vi "LabVIEW+Suite Demo Station.vi"() -> ()   [LabVIEW 2020]
doc: "This template is for the Queued Message Handler design pattern.\n\nThe Event Handling Loop generates messages based on user interface actions.\n\nThe Message Handling Loop processes messages generated by the Event Handling Loop, or by other messages. The messages are string values, so new messages can be added easily to the Message Cases case structure in the Message Handling Loop. Each message cluster can also provide an optional value for Message Data, which is a variant that can be converted to whatever message-specific data is required."
uses:
  support/Demo_class/Demo.lvclass
  support/Demo_class/Demo.lvclass/Demo.ctl
  support/UI Data--cluster.ctl
  support/Message Queue/lvdemo_Message Queue.lvlib
  support/Message Queue/Enqueue Message (Single).vi
  support/Configuration--cluster.ctl
  support/Tree Tag to Demo--map.ctl
panel:
  out "Title Text":string
  in  "Favorites Ring":u16(ring) items=["All Features"]
  in  "Tree":string(tree)
  in  "Slideshow":bool
  in  "Back":bool
  in  "Try It":bool
  in  "Credits":string="The code for this demo station is available at bit.ly/labviewdemostation"
  in  "Forward":bool
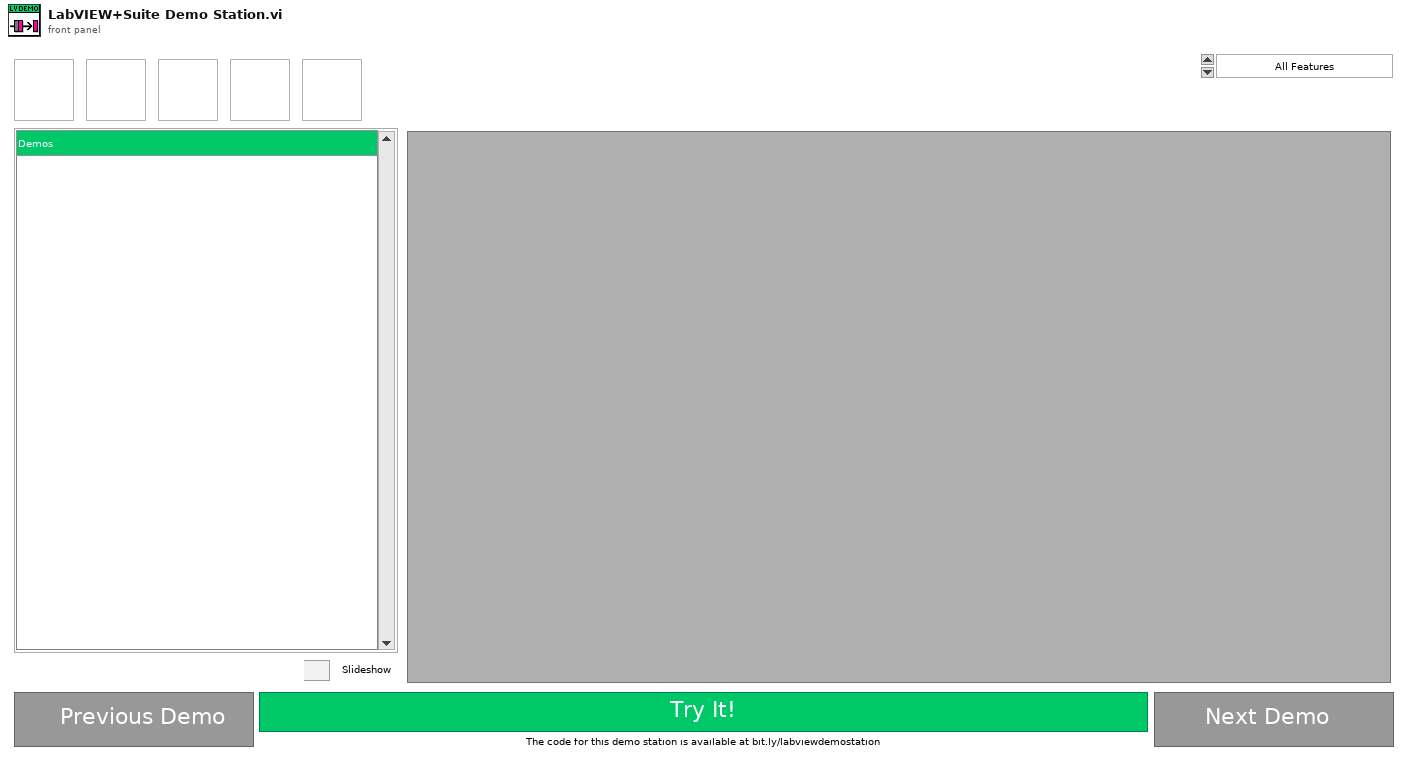
[diagram p1: front panel]
types:
  T1 = typedef "UI Data--cluster.ctl" = cluster{"Configuration":T2, "Start Timestamp":dbl, "Active Demos":T3, "Available Demos":T3}
  T2 = typedef "Configuration--cluster.ctl" = cluster{"Window Title":string, "Start Maximized":bool, "Slide Duration":i32, "Ignored Demos":string[], "Top Level Folder Order":string[], "Favorites":map{string, string[]}}
  T3 = typedef "Tree Tag to Demo--map.ctl" = map{string, refnum<class "Demo.lvclass">}
  T4 = typedef "lvdemo_Message Queue.lvlib/All Message Queues.ctl" = cluster{"UI":refnum<queue>}
  T5 = typedef "eventvkey.ctl" = enum16{"ASCII", "Enter", "Return", "Shift", "Ctrl", "Alt", "Cmd", "Opt", "Caps", "NumLock", "Clear", "Break", "Up", "Down", "Left", "Right", "Insert", "Delete", "Home", "End", "PageUp", "PageDown", "Escape", "Help", "Pause", "ScrollLock", "F1", "F2", "F3", "F4", "F5", "F6", "F7", "F8", "F9", "F10", "F11", "F12", "F13", "F14", "F15", "F16", "F17", "F18", "F19", "F20", "F21", "F22", "F23", "F24", "Play", "VolumeUp", "VolumeDown", "Mute", "Two Byte Char"}
  T6 = enum32{"Invalid", "Standard", "Closed", "Hidden", "Minimized", "Maximized"}
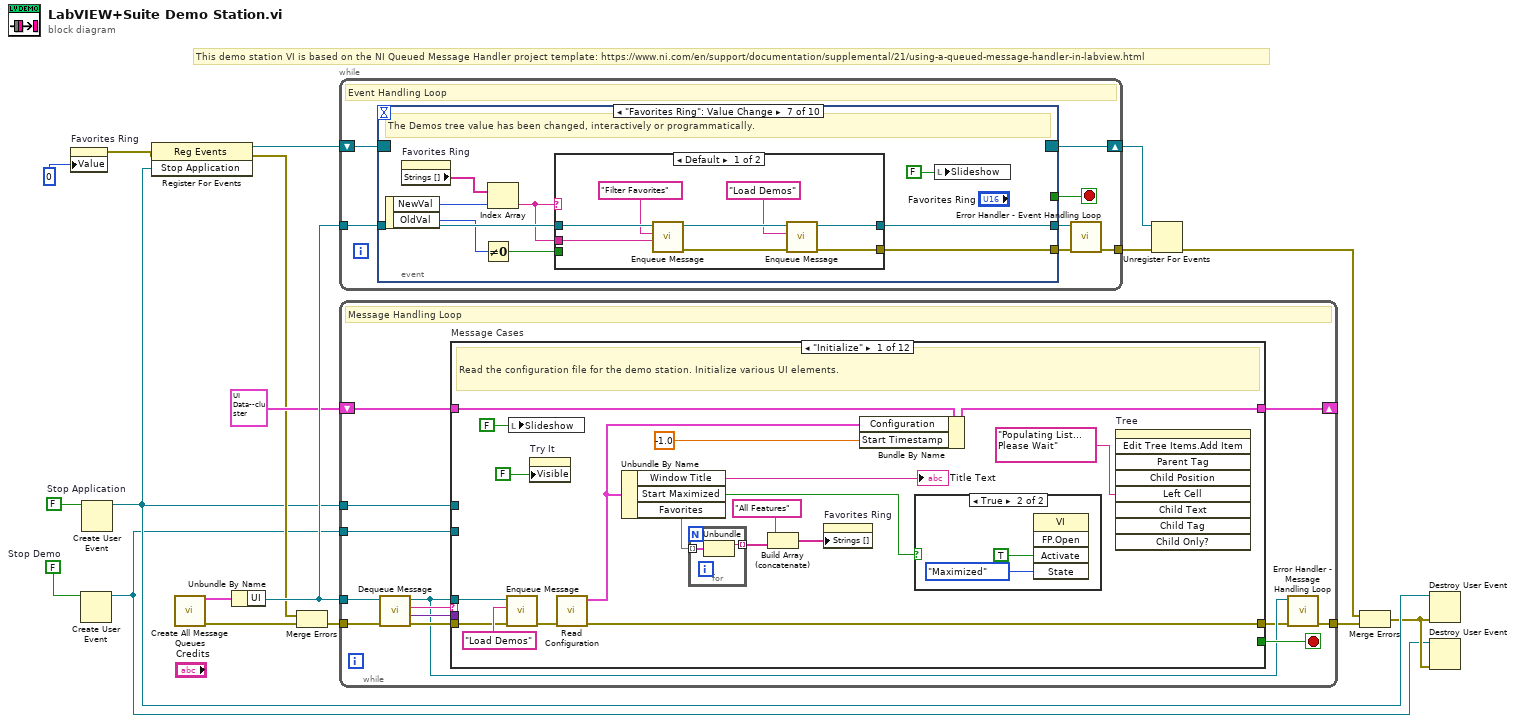
[diagram p0: block diagram]
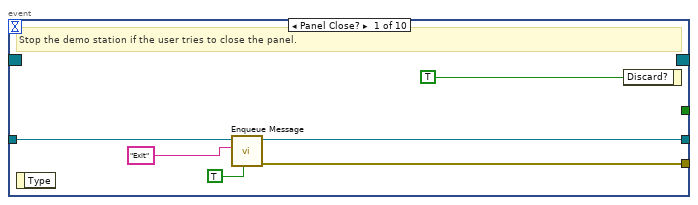
[diagram p2: hidden frame]
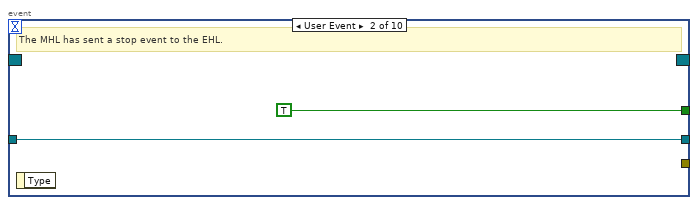
[diagram p3: hidden frame]
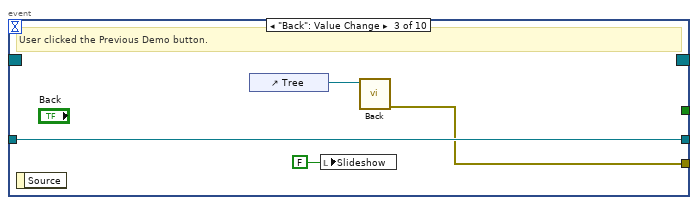
[diagram p4: hidden frame]
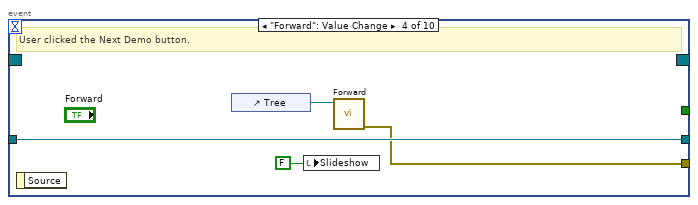
[diagram p5: hidden frame]
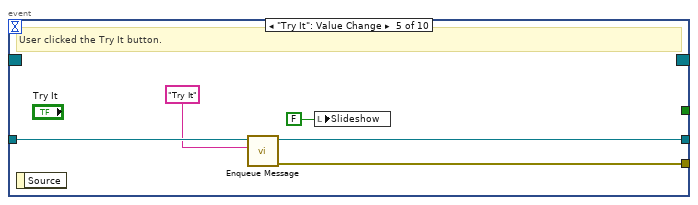
[diagram p6: hidden frame]
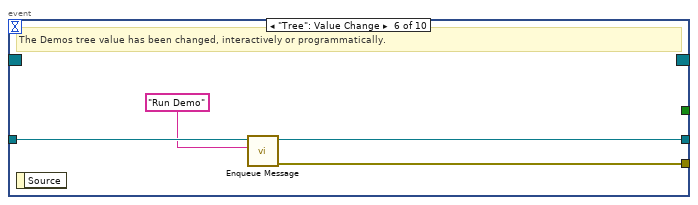
[diagram p7: hidden frame]
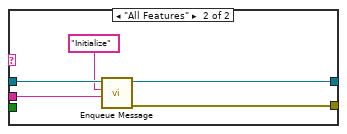
[diagram p8: hidden frame]
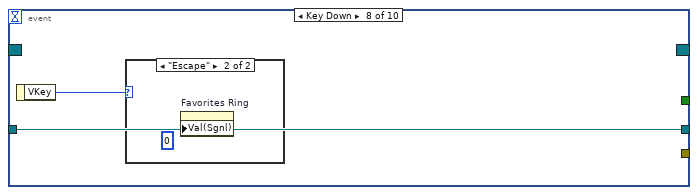
[diagram p9: hidden frame]
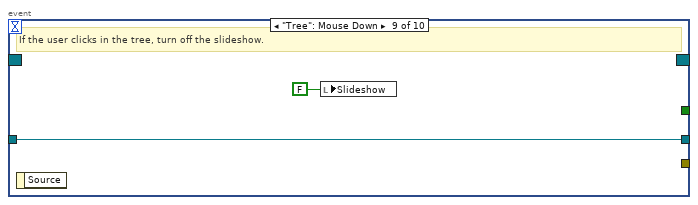
[diagram p11: hidden frame]
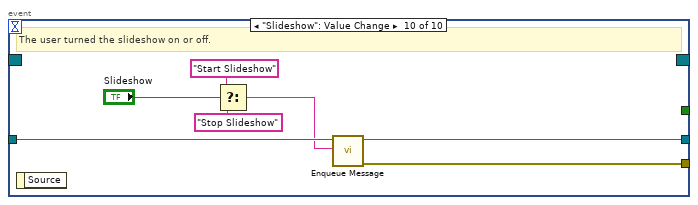
[diagram p12: hidden frame]
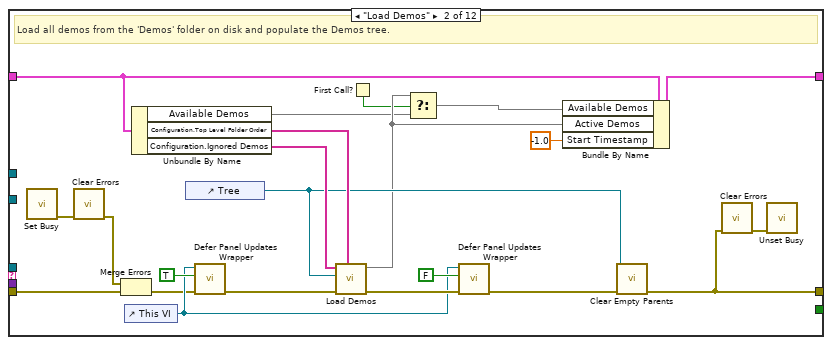
[diagram p14: hidden frame]
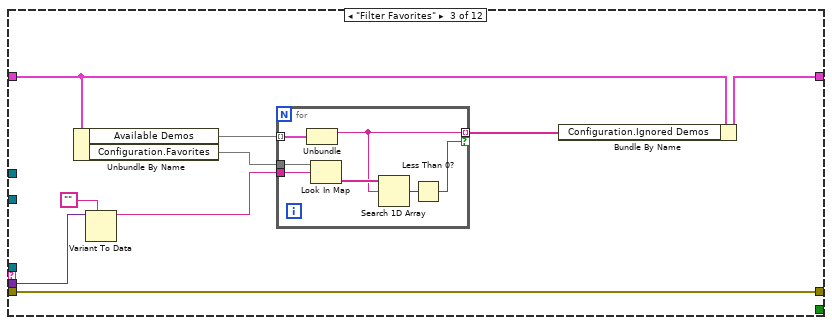
[diagram p15: hidden frame]
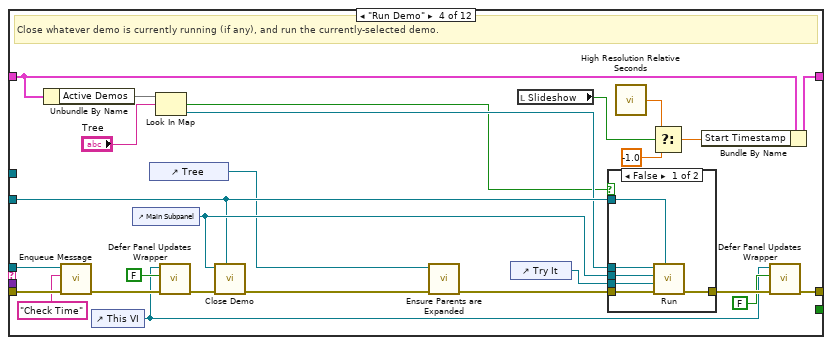
[diagram p16: hidden frame]
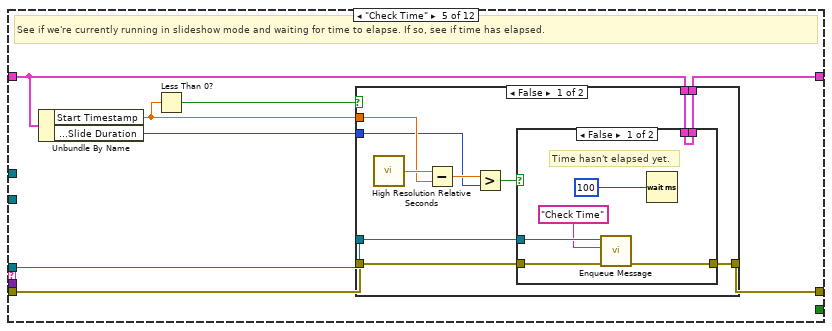
[diagram p18: hidden frame]
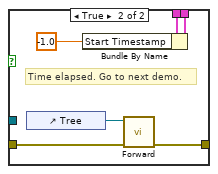
[diagram p19: hidden frame]
diagram:
  w5 = FALSE  # Stop Demo
  w7 = FALSE  # Stop Application
  # "This demo station VI is based on the NI Queued Message Handler project template: https://www.ni.com/en/support/documentation/supplemental/21/using-a-queued-message-handler-in-labview.html"
  n1 = property on="Favorites Ring" class="Ring (strict)"("Value"=u16 0 ("Value (Signaling)")) -> (error out=w1:errorcluster)  [unwired: 2 in, 1 out]
  n2 = Create User Event(user event datatype=w5) -> (user event=w3:refnum<user-event>)  [unwired: 1 in, 1 out]
  n3 = Create User Event(user event datatype=w7) -> (user event=w6:refnum<user-event>)  [unwired: 1 in, 1 out]
  n4 = register-events(error in=w1, w6) -> (reference out=w10:refnum<event-registration>, error out=w8:errorcluster)  [unwired: 1 in]
  n5 = call "Create All Message Queues.vi"() -> ("error out"=w18:errorcluster, "Message Queues out"=w17:T4)  [unwired: 10 in]
  n6 = Unbundle By Name(w17) -> ("UI"=w15:refnum<queue>)
  n7 = Merge Errors(w8, w18) -> (w9:errorcluster)
  n8 = while {
    tunnel: w15 -> [w25]
    shift-right: [w23] -> w13
    shift-left: w10 -> [w24]
    tunnel: [w19] -> w11
    stop <- w21 stop-if-true
    # "Event Handling Loop"
    n9 = event shown="[6] \"Favorites Ring\": Value Change" {
      selector: w24 -> [_ _ _ _ _ _ _ _ _ _]
      dyn-events: [_ _ _ _ _ _ _ _ _ _] -> w23
      timeout: _ -> [_ _ _ _ _ _ _ _ _ _]
      tunnel: [_ TRUE ("Discard?") _ _ _ _ _ _ _ _] -> w21
      tunnel: w25 -> [w30 w33 w37 w41 w46 w50 w59 w74 w77 w84]
      tunnel: [w29 _ w35 w39 w44 w48 w58 _ _ w80] -> w22
      tunnel: [w28 w33 w37 w41 w45 w49 w57 w74 w77 w81] -> w20
      event Panel Close? {
        # "Stop the demo station if the user tries to close the panel."
        n10 = event-data() -> ()  [unwired: 1 in, 1 out]
        n11 = call-poly "Enqueue Message.vi"("Priority Message? (F)"=TRUE, "Message"="Exit", "Message Queue"=w30) -> ("error out"=w29:errorcluster, "dup Message Queue"=w28:refnum<queue>)  [unwired: 7 in]
        n12 = event-data("Discard?"=TRUE) -> ()  [unwired: 1 in, 1 out]
      }
      event User Event {
        # "The MHL has sent a stop event to the EHL."
        n13 = event-data() -> ()  [unwired: 1 in, 1 out]
      }
      event "Back": Value Change {
        # "User clicked the Previous Demo button."
        n14 = event-data() -> ()  [unwired: 1 in, 1 out]
        n15 = control-ref of="Tree"() -> (w36:refnum<vi>)
        n16 = local write "Slideshow"(FALSE ("Slideshow")) -> ()
        n17 = call "Back.vi"("Tree"=w36) -> ("error out"=w35:errorcluster)  [unwired: 10 in]
      }
      event "Forward": Value Change {
        # "User clicked the Next Demo button."
        n18 = event-data() -> ()  [unwired: 1 in, 1 out]
        n19 = control-ref of="Tree"() -> (w40:refnum<vi>)
        n20 = local write "Slideshow"(FALSE ("Slideshow")) -> ()
        n21 = call "Forward.vi"("Tree"=w40) -> ("error out"=w39:errorcluster)  [unwired: 10 in]
      }
      event "Try It": Value Change {
        # "User clicked the Try It button."
        n22 = event-data() -> ()  [unwired: 1 in, 1 out]
        n23 = call-poly "Enqueue Message.vi"("Message"="Try It", "Message Queue"=w46) -> ("error out"=w44:errorcluster, "dup Message Queue"=w45:refnum<queue>)  [unwired: 8 in]
        n24 = local write "Slideshow"(FALSE ("Slideshow")) -> ()
      }
      event "Tree": Value Change {
        # "The Demos tree value has been changed, interactively or programmatically."
        n25 = event-data() -> ()  [unwired: 1 in, 1 out]
        n26 = call-poly "Enqueue Message.vi"("Message"="Run Demo", "Message Queue"=w50) -> ("error out"=w48:errorcluster, "dup Message Queue"=w49:refnum<queue>)  [unwired: 8 in]
      }
      event "Favorites Ring": Value Change {
        # "The Demos tree value has been changed, interactively or programmatically."
        n27 = event-data() -> ("NewVal"=w54:u16, "OldVal"=w52:u16)  [unwired: 1 in]
        n28 = property on="Favorites Ring" class="Ring (strict)"() -> ("Strings []"=w55:string[])  [unwired: 2 in, 2 out]
        n29 = Not Equal To 0?(x=w52) -> (x != 0?=w51:bool)
        n30 = Index Array(array=w55, index=w54) -> (element=w53:string)
        n31 = case shown="Default" w53 {
          tunnel: w59 -> [w61 w72]
          tunnel: [w65 w69] -> w58
          tunnel: [w64 w70] -> w57
          tunnel: w53 -> [w62 w68]
          tunnel: w51 -> [_ _]
          frame Default {
            n32 = call-poly "Enqueue Message.vi"("Message Data"=w62, "Message"="Filter Favorites", "Message Queue"=w61) -> ("error out"=w66:errorcluster, "dup Message Queue"=w67:refnum<queue>)  [unwired: 7 in]
            n33 = call-poly "Enqueue Message.vi"("error in (no error)"=w66, "Message"="Load Demos", "Message Queue"=w67) -> ("error out"=w65:errorcluster, "dup Message Queue"=w64:refnum<queue>)  [unwired: 7 in]
          }
          frame "All Features" {
            n34 = call-poly "Enqueue Message.vi"("Message Data"=w68, "Message"="Initialize", "Message Queue"=w72) -> ("error out"=w69:errorcluster, "dup Message Queue"=w70:refnum<queue>)  [unwired: 7 in]
          }
        }
        n35 = local write "Slideshow"(FALSE ("Slideshow")) -> ()
      }
      event Key Down {
        n36 = event-data() -> ("VKey"=w73:T5)  [unwired: 1 in]
        n37 = case shown="\"Escape\"" w73 {
          frame "ASCII", Default {
          }
          frame "Escape" {
            n38 = property on="Favorites Ring" class="Ring (strict)"("Val(Sgnl)"=u16 0 ("Value (Signaling)")) -> ()  [unwired: 2 in, 2 out]
          }
        }
      }
      event "Tree": Mouse Down {
        # "If the user clicks in the tree, turn off the slideshow."
        n39 = event-data() -> ()  [unwired: 1 in, 1 out]
        n40 = local write "Slideshow"(FALSE ("Slideshow")) -> ()
      }
      event "Slideshow": Value Change {
        # "The user turned the slideshow on or off."
        n41 = event-data() -> ()  [unwired: 1 in, 1 out]
        n42 = Select(t="Start Slideshow", s="Slideshow", f="Stop Slideshow") -> (s? t:f=w78:string)
        n43 = call-poly "Enqueue Message.vi"("Message"=w78, "Message Queue"=w84) -> ("error out"=w80:errorcluster, "dup Message Queue"=w81:refnum<queue>)  [unwired: 8 in]
      }
    }
    n44 = call "Error Handler - Event Handling Loop.vi"("error in (no error)"=w22, "Message Queue"=w20) -> ("dup error in"=w19:errorcluster)  [unwired: 8 in, 1 out]
  }
  n45 = while {
    tunnel: w15 -> [w89]
    shift-right: [w96] -> _
    shift-left: T1 {"Configuration"={"Window Title"="", "Start Maximized"=FALSE, "Slide Duration"=0, "Ignored Demos"=[], "Top Level Folder Order"=[], "Favorites"={}}, "Start Timestamp"=0.0, "Active Demos"={}, "Available Demos"={}} ("Data Cluster") -> [w97]
    tunnel: w6 -> [w94]
    tunnel: w9 -> [w93]
    tunnel: [w87] -> w16
    tunnel: w3 -> [w85]
    stop <- w95 stop-if-true
    # "Message Handling Loop"
    n46 = call "Dequeue Message.vi"("error in (no error)"=w93, "Message Queue"=w89) -> ("error out"=w92:errorcluster, "Message Data"=w90:variant, "Message"=w91:string, "dup Message Queue"=w88:refnum<queue>)  [unwired: 6 in]
    n47 = case "Message Cases" shown="\"Initialize\"" w91 {
      selector: w91 -> [_ _ _ _ _ _ _ _ _ _ _ w277]
      tunnel: w88 -> [w110 _ _ w182 w195 _ _ _ _ _ w270 _]
      tunnel: w92 -> [w108 w138 w150 w183 w194 w226 w235 w241 w248 w251 w266 _]
      tunnel: [w106 w125 w150 w169 w193 w227 w234 w241 w242 w249 w267 w274] -> w86
      tunnel: w97 -> [w115 w127 w149 w178 w191 w230 w236 w240 w247 w250 w261 w280]
      tunnel: [w114 w141 w143 w177 w192 w232 w236 w239 w247 w250 w261 w280] -> w96
      tunnel: [_ _ _ _ _ _ _ _ _ _ TRUE _] -> w95
      tunnel: w90 -> [_ _ w146 _ _ _ _ _ w246 _ w263 _]
      tunnel: w94 -> [_ _ _ _ _ _ _ _ _ _ w259 _]
      tunnel: w85 -> [_ _ _ w176 _ _ _ _ _ _ w256 _]
      frame "Initialize" {
        # "Read the configuration file for the demo station. Initialize various UI elements."
        n48 = call-poly "Enqueue Message.vi"("error in (no error)"=w108, "Message"="Load Demos", "Message Queue"=w110) -> ("error out"=w107:errorcluster)  [unwired: 7 in, 1 out]
        n49 = local write "Slideshow"(FALSE ("Demo Mode")) -> ()
        n50 = property on="Try It" class="Bool"("Visible"=FALSE) -> ()  [unwired: 2 in, 2 out]
        n51 = call "Read Configuration.vi"("error in"=w107) -> ("error out"=w106:errorcluster, "Configuration"=w113:T2)  [unwired: 9 in]
        n52 = Unbundle By Name(w113) -> ("Window Title"=→"Title Text":string, "Start Maximized"=w111:bool, "Favorites"=w101:map{string, string[]})
        n53 = for {
          tunnel: w101 -> [w117] mode=indexing
          tunnel: [w116] -> w100 mode=indexing
          n54 = Unbundle(w117) -> ("key"=w116:string)  [unwired: 1 out]
        }
        n55 = Build Array (concatenate)("All Features", w100) -> (w98:string[])
        n56 = property on="Favorites Ring" class="Ring (strict)"("Strings []"=w98) -> ()  [unwired: 2 in, 2 out]
        n57 = Bundle By Name(cluster=w115, "Configuration"=w113, "Start Timestamp"=-1.0) -> (w114:T1)
        n58 = case shown="True" w111 {
          frame False {
          }
          frame True {
            n59 = invoke class="VI" method="FP.Open"("Activate"=TRUE ("Activate?"), "State"=T6."Maximized") -> ()  [unwired: 3 in, 5 out]
          }
        }
        n60 = invoke on="Tree" class="Tree (strict)" method="Edit Tree Items.Add Item"("Left Cell"="Populating List... Please Wait") -> ()  [unwired: 8 in, 9 out]
      }
      frame "Load Demos" {
        # "Load all demos from the 'Demos' folder on disk and populate the Demos tree."
        n61 = call <vilib>:"Set Busy.vi"() -> ("error out"=w132:errorcluster)  [unwired: 10 in, 1 out]
        n62 = call <vilib>:"Clear Errors.vi"("error in (no error)"=w132) -> ("error out"=w130:errorcluster)  [unwired: 5 in, 1 out]
        n63 = Merge Errors(w130, w138) -> (w131:errorcluster)
        n64 = control-ref of="This VI"() -> (w133:refnum<vi>)
        n65 = Unbundle By Name(w127) -> ("Available Demos"=w122:T3, "Configuration.Top Level Folder Order"=w128:string[], "Configuration.Ignored Demos"=w139:string[])
        n66 = control-ref of="Tree"() -> (w124:refnum<vi>)
        n67 = call "Defer Panel Updates Wrapper.vi"("error in"=w131, "Defer Updates"=TRUE, "VI"=w133) -> ("error out"=w137:errorcluster)  [unwired: 8 in]
        n68 = call "Load Demos.vi"("Top Level Folder Order"=w128, "error in"=w137, "Tree"=w124, "Ignored Demos"=w139) -> ("error out"=w136:errorcluster, "Demos"=w123:T3)  [unwired: 6 in]
        n69 = First Call?() -> (First Call?: T/F=w120:bool)
        n70 = Select(t=w123, s=w120, f=w122) -> (s? t:f=w121:T3)
        n71 = call "Defer Panel Updates Wrapper.vi"("error in"=w136, "Defer Updates"=FALSE, "VI"=w133) -> ("error out"=w126:errorcluster)  [unwired: 8 in]
        n72 = Bundle By Name(cluster=w127, "Available Demos"=w121, "Active Demos"=w123, "Start Timestamp"=-1.0) -> (w141:T1)
        n73 = call "Clear Empty Parents.vi"("error in (no error)"=w126, "TreeControl in"=w124) -> ("error IO"=w125:errorcluster)  [unwired: 9 in]
        n74 = call <vilib>:"Clear Errors.vi"("error in (no error)"=w125) -> ("error out"=w129:errorcluster)  [unwired: 5 in, 1 out]
        n75 = call <vilib>:"Unset Busy.vi"("error in (no error)"=w129) -> ()  [unwired: 10 in, 1 out]
      }
      frame "Filter Favorites" {
        n76 = Unbundle By Name(w149) -> ("Available Demos"=w148:T3, "Configuration.Favorites"=w147:map{string, string[]})
        n77 = Variant To Data(type="", Variant=w146) -> (data=w144:string)  [unwired: 1 in, 1 out]
        n78 = for {
          tunnel: w148 -> [w157] mode=indexing
          tunnel: w147 -> [w156]
          tunnel: w144 -> [w155]
          tunnel: [w152] -> w142 mode=indexing if=w151
          n79 = Unbundle(w157) -> ("Tree Tag"=w152:string)  [unwired: 1 out]
          n80 = Look In Map(map=w156, key=w155) -> (value=w154:string[])  [unwired: 1 in, 1 out]
          n81 = Search 1D Array(1D array=w154, element=w152) -> (index of element=w153:i32)  [unwired: 1 in]
          n82 = Less Than 0?(x=w153) -> (x < 0?=w151:bool)
        }
        n83 = Bundle By Name(cluster=w149, "Configuration.Ignored Demos"=w142) -> (w143:T1)
      }
      frame "Run Demo" {
        # "Close whatever demo is currently running (if any), and run the currently-selected demo."
        n84 = Unbundle By Name(w178) -> ("Active Demos"=w175:T3)
        n85 = call-poly "Enqueue Message.vi"("error in (no error)"=w183, "Message"="Check Time", "Message Queue"=w182) -> ("error out"=w172:errorcluster)  [unwired: 7 in, 1 out]
        n86 = control-ref of="This VI"() -> (w166:refnum<vi>)
        n87 = control-ref of="Main Subpanel"() -> (w181:refnum<vi>)
        n88 = control-ref of="Tree"() -> (w162:refnum<vi>)
        n89 = Look In Map(map=w175, key="Tree") -> (key not found?=w165:bool, value=w173:refnum<class "Demo.lvclass">)  [unwired: 1 in]
        n90 = call "Defer Panel Updates Wrapper.vi"("error in"=w172, "Defer Updates"=FALSE, "VI"=w166) -> ("error out"=w171:errorcluster)  [unwired: 8 in]
        n91 = call "Close Demo.vi"("Stop Demo"=w176, "error in"=w171, "Main Subpanel"=w181) -> ("error out"=w164:errorcluster)  [unwired: 8 in]
        n92 = call "Ensure Parents are Expanded.vi"("error in"=w164, "Tree"=w162) -> ("error out"=w163:errorcluster)  [unwired: 9 in]
        n93 = control-ref of="Try It"() -> (w179:refnum<vi>)
        n94 = local read "Slideshow"() -> (w159:bool)
        n95 = case shown="False" w165 {
          tunnel: w163 -> [w189 w190]
          tunnel: w181 -> [w188 _]
          tunnel: w179 -> [w187 _]
          tunnel: w176 -> [w186 _]
          tunnel: w173 -> [w185 _]
          tunnel: [w184 w190] -> w170
          frame False {
            n96 = call-dynamic "Run.vi"("Stop Demo"=w186, "error in"=w189, "Try It Button"=w187, "Main Subpanel"=w188, "Demo in"=w185) -> ("error out"=w184:errorcluster)  [unwired: 5 in, 1 out]
          }
          frame True {
          }
        }
        n97 = call <vilib>:"High Resolution Relative Seconds.vi"() -> ("relative seconds"=w161:dbl)
        n98 = Select(t=w161, s=w159, f=-1.0) -> (s? t:f=w160:dbl)
        n99 = Bundle By Name(cluster=w178, "Start Timestamp"=w160) -> (w177:T1)
        n100 = call "Defer Panel Updates Wrapper.vi"("error in"=w170, "Defer Updates"=FALSE, "VI"=w166) -> ("error out"=w169:errorcluster)  [unwired: 8 in]
      }
      frame "Check Time" {
        # "See if we're currently running in slideshow mode and waiting for time to elapse. If so, see if time has elapsed."
        n101 = Unbundle By Name(w191) -> ("Start Timestamp"=w197:dbl, "Configuration.Slide Duration"=w196:i32)
        n102 = Less Than 0?(x=w197) -> (x < 0?=w198:bool)
        n103 = case shown="False" w198 {
          tunnel: w197 -> [w207 _]
          tunnel: w196 -> [w205 _]
          tunnel: w195 -> [w202 _]
          tunnel: w194 -> [w204 w222]
          tunnel: [w203 w222] -> w193
          tunnel: w191 -> [w200 w221]
          tunnel: [w199 w221] -> w192
          frame False {
            n104 = call <vilib>:"High Resolution Relative Seconds.vi"() -> ("relative seconds"=w208:dbl)
            n105 = Subtract(x=w208, y=w207) -> (x-y=w206:dbl)
            n106 = Greater?(x=w206, y=w205) -> (0:w201:bool)
            n107 = case shown="False" w201 {
              tunnel: w204 -> [w213 w216]
              tunnel: [w212 w217] -> w203
              tunnel: w202 -> [w211 _]
              tunnel: w200 -> [w209 w220]
              tunnel: [w209 w219] -> w199
              frame False {
                # "Time hasn't elapsed yet."
                n108 = call-poly "Enqueue Message.vi"("error in (no error)"=w213, "Message"="Check Time", "Message Queue"=w211) -> ("error out"=w212:errorcluster)  [unwired: 7 in, 1 out]
                n109 = Wait (ms)(milliseconds to wait=u32 100) -> ()  [unwired: 1 out]
              }
              frame True {
                # "Time elapsed. Go to next demo."
                n110 = control-ref of="Tree"() -> (w215:refnum<vi>)
                n111 = Bundle By Name(cluster=w220, "Start Timestamp"=-1.0) -> (w219:T1)
                n112 = call "Forward.vi"("error in"=w216, "Tree"=w215) -> ("error out"=w217:errorcluster)  [unwired: 9 in]
              }
            }
          }
          frame True {
            # "No timestamp stored, don't check"
          }
        }
      }
      frame "Try It" {
        # "Execute the 'Try It' code for the current demo."
        n113 = Unbundle By Name(w230) -> ("Active Demos"=w229:T3)
        n114 = local read "Tree"() -> (w228:string)
        n115 = Look In Map(map=w229, key=w228) -> (value=w225:refnum<class "Demo.lvclass">)  [unwired: 1 in, 1 out]
        n116 = control-ref of="This VI"() -> (w224:refnum<vi>)
        n117 = call "Try It.vi"("error in"=w226, "Main Demo UI"=w224, "Demo"=w225) -> ("error out"=w227:errorcluster)  [unwired: 8 in]
        n118 = local write "Slideshow"(FALSE ("Slideshow")) -> ()
        n119 = Bundle By Name(cluster=w230, "Start Timestamp"=-1.0) -> (w232:T1)
      }
      frame "Start Slideshow" {
        # "Start the slideshow."
        n120 = control-ref of="Tree"() -> (w233:refnum<vi>)
        n121 = call "Forward.vi"("error in"=w235, "Tree"=w233) -> ("error out"=w234:errorcluster)  [unwired: 9 in]
      }
      frame "Stop Slideshow" {
        # "Stop slideshow."
        n122 = Bundle By Name(cluster=w240, "Start Timestamp"=-1.0) -> (w239:T1)
        n123 = local write "Slideshow"(FALSE ("Slideshow")) -> ()
      }
      frame "Error" {
        # "Display an error dialog. This message is sent by the \"Error Handler\" VIs at the end of other loops in this application."
        n124 = Variant To Data(error in=w248, type=errorcluster {"status"=FALSE, "code"=0, "source"=""} ("error constant"), Variant=w246) -> (data=w244:errorcluster, error out=w243:errorcluster)
        n125 = call <vilib>:"Simple Error Handler.vi"("error in (no error)"=w244) -> ()  [unwired: 4 in, 5 out]
        n126 = Merge Errors(w243) -> (w242:errorcluster)
      }
      frame "---Copy This Frame---" {
        # "Duplicate this frame when creating new messages.  Change this comment in the duplicated frame to describe this message."
        n127 = Merge Errors(w251) -> (w249:errorcluster)
      }
      frame "Exit" {
        # "Restore to non-maximized to avoid weird front panel redraw issues."
        # "Empty tree on close"
        # "Stop the VI"
        # "Exit - Exit the application."
        n128 = Variant To Data(type=errorcluster {"status"=FALSE, "code"=0, "source"=""} ("error constant"), Variant=w263) -> (data=w264:errorcluster)  [unwired: 1 in, 1 out]
        n129 = Generate User Event(user event=w259, event data cluster=TRUE ("event data")) -> ()  [unwired: 2 in, 2 out]
        n130 = Unbundle By Name(w261) -> ("Active Demos"=w260:T3)
        n131 = call <vilib>:"Simple Error Handler.vi"("error in (no error)"=w264) -> ()  [unwired: 4 in, 5 out]
        n132 = Release Queue(queue=w270, error in (no error)=w266) -> (error out=w268:errorcluster)  [unwired: 1 in, 2 out]
        n133 = Generate User Event(user event=w256, event data cluster=TRUE ("event data")) -> (error out=w257:errorcluster)  [unwired: 2 in, 1 out]
        n134 = for {
          tunnel: w260 -> [w273] mode=indexing
          tunnel: w257 -> [_]
          n135 = Unbundle(w273) -> ("Demo"=w271:refnum<class "Demo.lvclass">)  [unwired: 1 out]
          n136 = property class="Demo"(reference=w271) -> ("Accessors:VI"=w272:refnum<vi>)  [unwired: 1 in, 2 out]
          n137 = Close Reference(reference=w272) -> ()  [unwired: 1 in, 1 out]
        }
        n138 = Merge Errors(w257, w268) -> (w267:errorcluster)
        n139 = invoke on="Tree" class="Tree (strict)" method="Edit Tree Items.Delete"("tag"="", "Delete Children"=TRUE) -> ()  [unwired: 3 in, 5 out]
        n140 = invoke class="VI" method="FP.Open"("Activate"=TRUE ("Activate?"), "State"=T6."Standard") -> ()  [unwired: 3 in, 5 out]
      }
      frame Default {
        # "'Default' case only runs if there is a message that isn't defined in any of the other cases.  Output a programming error."
        n141 = Format Into String(format string="The invalid message string \"%s\" was received in the Message Handling Loop.", w277) -> (resulting string=w275:string)  [unwired: 2 in, 1 out]
        n142 = call <vilib>:"Error Cluster From Error Code.vi"("show call chain? (False)"=TRUE, "error message (\"\")"=w275, "error code (0)"=1) -> ("error out"=w274:errorcluster)  [unwired: 6 in]
      }
    }
    n143 = call "Error Handler - Message Handling Loop.vi"("error in (no error)"=w86, "Message Queue"=w88) -> ("dup error in"=w87:errorcluster)  [unwired: 8 in, 1 out]
  }
  n144 = Unregister For Events(event registration refnum=w13, error in=w11) -> (error out=w14:errorcluster)
  n145 = Merge Errors(w14, w16) -> (w4:errorcluster)
  n146 = Destroy User Event(user event=w6, error in=w4) -> ()  [unwired: 1 out]
  n147 = Destroy User Event(user event=w3, error in=w4) -> ()  [unwired: 1 out]
